vi "scan.vi"(8 "error in (no error)":errorcluster, 11 "Input":string="34,45,89") -> (0 "error out":errorcluster, 3 "Output":string)   [LabVIEW 2014]
uses:
  <userlib>/Nanonis Prog Interface V5/Nanonis Prog Interface.lvlib
panel:
  in  "Channel":u8(ring)=14 items=["Current"=0, "Z (m)"=14]
  in  "Direction: Fwd/Bwd (T=Fwd)":bool=TRUE
  in  "milliseconds to wait":u32=3000
  in  "Angle (deg)":sgl=nan caption="Angle (deg) (NaN=no change)" format="%.2f"
  in  "Size (m)":cluster{"Width":sgl, "Height":sgl}={"Width"=1e-08, "Height"=1e-08} caption="Size (m) (NaN=no change)" {"Height" format="%.2p"; "Width" format="%.2p"}
  out "size(s)":i32=3
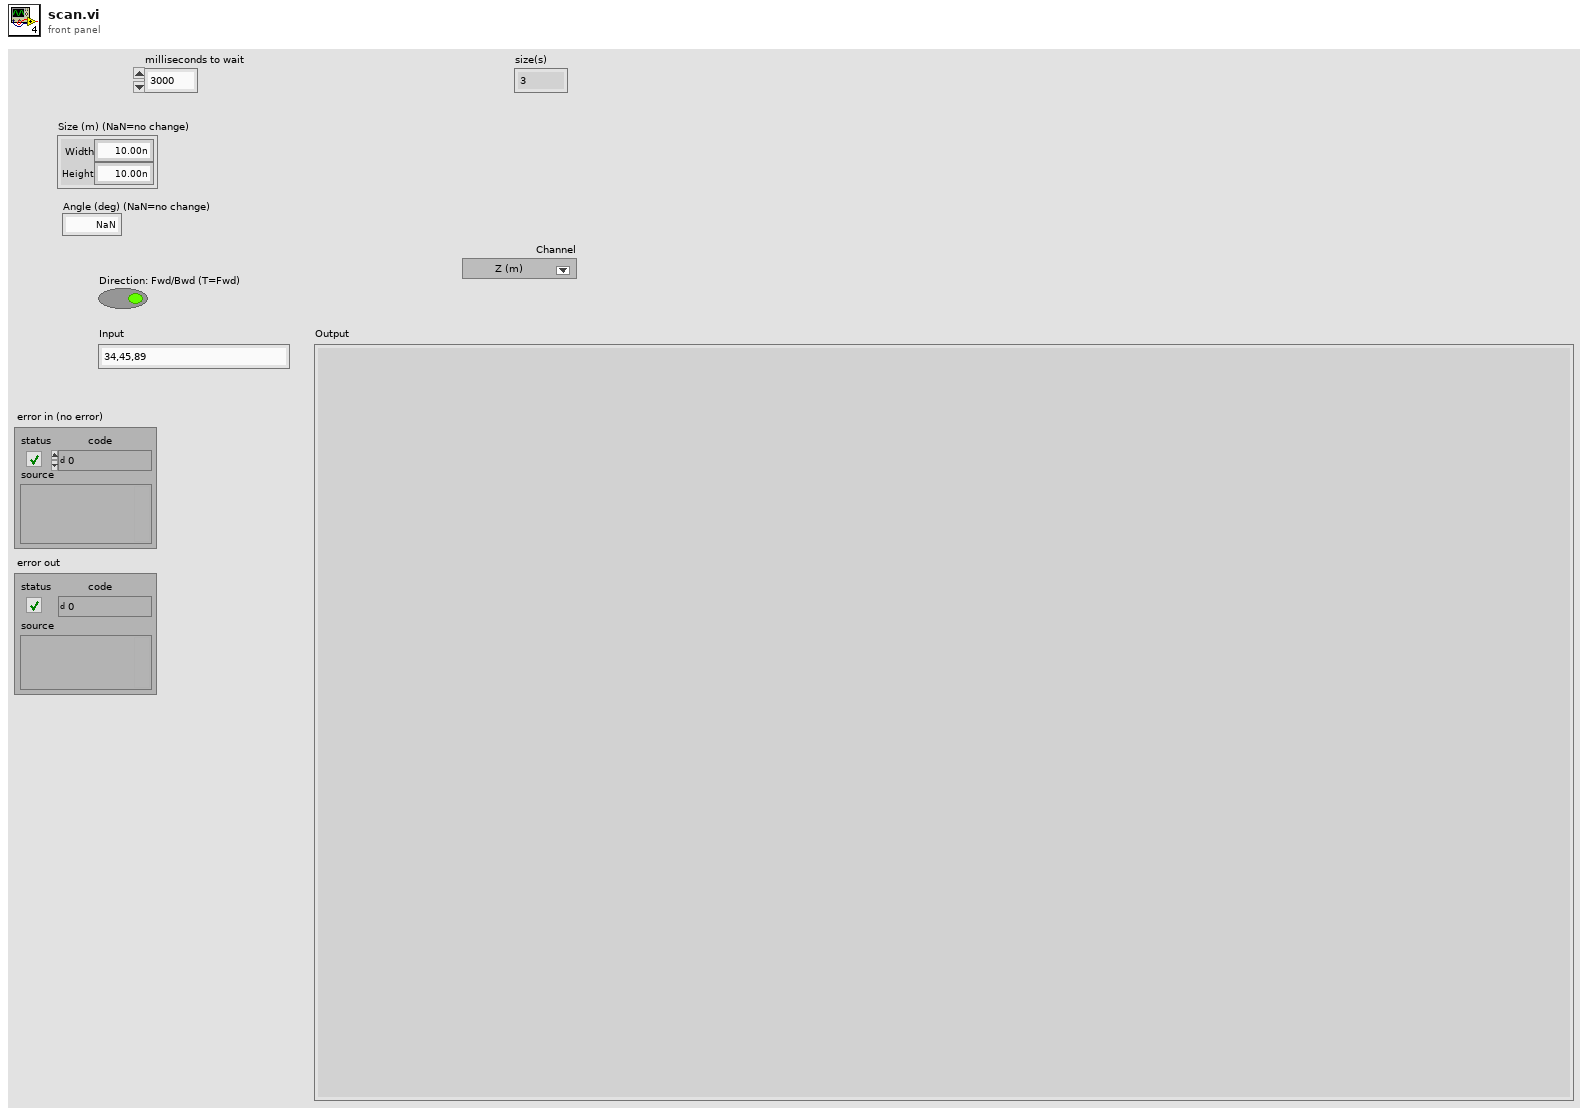
[diagram p1: front panel]
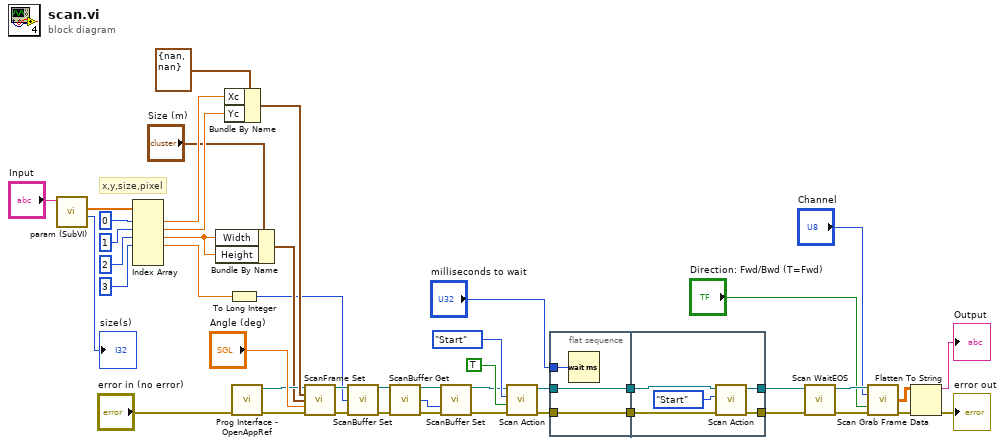
[diagram p0: block diagram]
diagram:
  # "x,y,size,pixel"
  n1 = call <userlib>:"param (SubVI).vi"("Input"="Input") -> ("num"=→"size(s)":i32, "parm"=w44:dbl[])  [unwired: 8 in, 1 out]
  n2 = Index Array(array=w44, index #1=0 ("index"), index #2=1 ("index"), index #3=2 ("index"), index #4=3 ("index")) -> (element #1=w42:dbl, element #2=w41:dbl, element #3=w16:dbl, element #4=w14:dbl)  [unwired: 2 in, 2 out]
  n3 = Bundle By Name(cluster="Size (m)", "Width"=w16, "Height"=w16) -> (w15:cluster{"Width":sgl, "Height":sgl})
  n4 = Bundle By Name(cluster=cluster{"Xc":sgl, "Yc":sgl} {"Xc"=nan, "Yc"=nan} ("Center coordinates (m)"), "Xc"=w42, "Yc"=w41) -> (w40:cluster{"Xc":sgl, "Yc":sgl})
  n5 = To Long Integer(number=w14) -> (32bit integer=w13:i32)
  n6 = call <userlib>:"Prog Interface - OpenAppRef.vi"("Error in (no error)"="error in (no error)") -> ("Error out"=w28:errorcluster, "Application reference"=w29:refnum<vi>)  [unwired: 5 in]
  n7 = call <userlib>:"ScanFrame Set.vi"("Application ref in"=w29, "Center coordinates (m)"=w40, "Size (m)"=w15, "Angle (deg)"="Angle (deg)", "error in (no error)"=w28) -> ("Application ref out"=w38:refnum<vi>, "error out"=w37:errorcluster)  [unwired: 9 in]
  n8 = call <userlib>:"ScanBuffer Set.vi"("Application ref in"=w38, "Pixels"=w13, "error in (no error)"=w37) -> ("Application ref out"=w4:refnum<vi>, "error out"=w3:errorcluster)  [unwired: 11 in]
  n9 = call <userlib>:"ScanBuffer Get.vi"("Application ref in"=w4, "error in (no error)"=w3) -> ("Application ref out"=w6:refnum<vi>, "Pixels/line"=w7:i32, "error out"=w5:errorcluster)  [unwired: 9 in, 2 out]
  n10 = call <userlib>:"ScanBuffer Set.vi"("Application ref in"=w6, "Lines"=w7, "error in (no error)"=w5) -> ("Application ref out"=w2:refnum<vi>, "error out"=w1:errorcluster)  [unwired: 11 in]
  n11 = call <userlib>:"Scan Action.vi"("error in (no error)"=w1, "Direction: up/down (T=up)"=TRUE, "Scan action (Start)"=enum16{"Start", "Stop", "Pause", "Resume"}."Start", "Application ref in"=w2) -> ("error out"=w33:errorcluster, "Application ref out"=w34:refnum<vi>)  [unwired: 5 in]
  n12 = flat-sequence {
    tunnel: w34 -> [w48]
    tunnel: w33 -> [w47]
    tunnel: "milliseconds to wait" -> [w49]
    tunnel: [w48] -> w31
    tunnel: [w47] -> w30
    tunnel: w31 -> [w54]
    tunnel: w30 -> [w53]
    tunnel: [w51] -> w26
    tunnel: [w50] -> w25
    frame #0 {
      n13 = Wait (ms)(milliseconds to wait=w49) -> ()  [unwired: 1 out]
    }
    frame #1 {
      n14 = call <userlib>:"Scan Action.vi"("error in (no error)"=w53, "Scan action (Start)"=enum16{"Start", "Stop", "Pause", "Resume"}."Start", "Application ref in"=w54) -> ("error out"=w50:errorcluster, "Application ref out"=w51:refnum<vi>)  [unwired: 6 in]
    }
  }
  n15 = call <userlib>:"Scan WaitEOS.vi"("error in (no error)"=w25, "Application ref in"=w26) -> ("error out"=w22:errorcluster, "Application ref out"=w24:refnum<vi>)  [unwired: 5 in, 2 out]
  n16 = call <userlib>:"Scan Grab Frame Data.vi"("Application ref in"=w24, "Channel index (0-23)"="Channel", "Direction: Fwd/Bwd (T=Fwd)"="Direction: Fwd/Bwd (T=Fwd)", "error in (no error)"=w22) -> ("Scan frame data"=w8:sgl[][], "error out"=w12:errorcluster)  [unwired: 7 in, 3 out]
  n17 = Flatten To String(anything=w8, error in (no error)=w12) -> (data string=→"Output":string, error out=→"error out":errorcluster)  [unwired: 2 in, 1 out]
